vi "AWS IoT Button - Upload to S3 Bucket.vi"() -> ()   [LabVIEW 2015]
doc: "Demonstrates how to programmatically upload AWS IoT Button data to an S3 bucket."
uses:
  Core/HTTP Request/Region.ctl
  IoT/Topic Rule.ctl
  IoT/CloudWatch Alarm.ctl
  IoT/CloudWatch Metric.ctl
  IoT/DynamoDB.ctl
  IoT/DynamoDBv2.ctl
  IoT/Elasticsearch.ctl
  IoT/Firehose.ctl
  IoT/Kinesis.ctl
  IoT/Lambda.ctl
  IoT/Republish.ctl
  IoT/S3.ctl
  IoT/SNS.ctl
  IoT/SQS.ctl
  Core/HTTP Request/AWS Credentials.ctl
  IoT/IoT Session/IoT Session.lvclass
  IoT/NI_AWS_IoT.lvlib
  S3/Bucket/Bucket.lvclass
  Core/HTTP Request/HTTP Request.lvclass
panel:
  in  "Bucket Name":string
  in  "AWS IoT Button Serial Number":string
  in  "Region":T1
  in  "Secret Key":string
  in  "Access Key":string
  # "Overview: Demonstrates how to programmatically upload AWS IoT Button data to an S3 bucket.\nRequirements: NI Cloud Toolkit for AWS, a configured AWS IoT Button, and a registered Amazon AWS account\nInstructions:\n1. Specify the Access Key and Secret Key for your AWS account. You can create an account at http://aws.amazon.com.\n2. Make sure you already have an AWS IoT Button configured in the AWS IoT Management Console on the amazon website.\n3. Specify the Region under which your AWS IoT Button is configured.\n4. Specify the AWS IoT Button Serial Number.\n5. Specify the Bucket Name where you want to upload the AWS IoT Button data. Note: This bucket must already exist, and it must be in the same region as the AWS IoT Button.\n6. Run the VI.\n7. Click the AWS IoT Button. After the green light appears on the button, you can use the AWS S3 Management Console to see the button data appear as a new file in the specified S3 bucket."
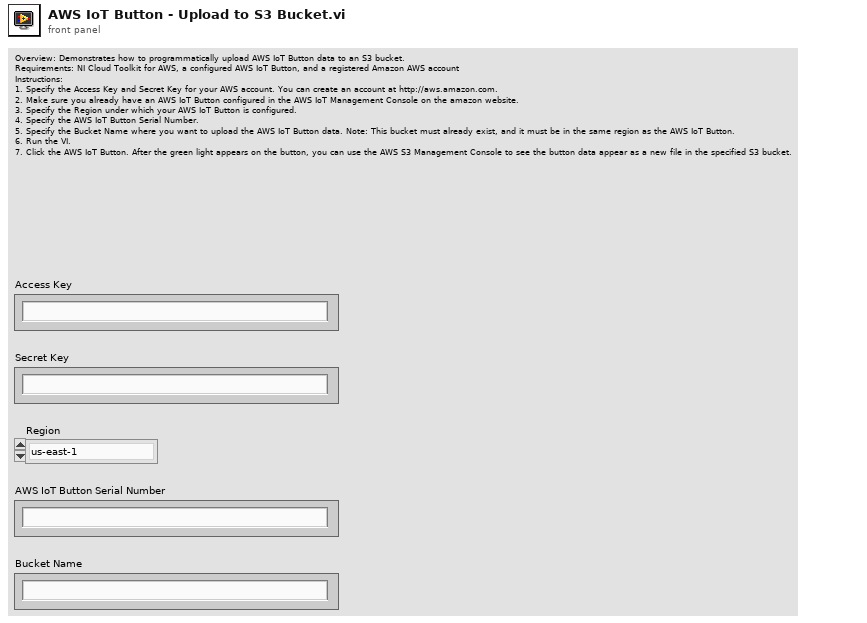
[diagram p1: front panel]
types:
  T1 = typedef "NI_AWS_Core.lvlib/HTTP Request.lvclass/Region.ctl" = enum16{"us-east-1", "us-east-2", "us-west-1", "us-west-2", "ap-northeast-1", "ap-northeast-2", "ap-southeast-1", "ap-southeast-2", "ca-central-1", "eu-central-1", "eu-west-1", "eu-west-2", "sa-east-1"}
  T2 = typedef "NI_AWS_Core.lvlib/HTTP Request.lvclass/AWS Credentials.ctl" = cluster{"Access Key":string, "Secret Key":string}
  T3 = typedef "NI_AWS_IoT.lvlib/S3.ctl" = cluster{"Bucket Name":string, "Canned ACL":string, "Key":string, "Role ARN":string}
  T4 = typedef "NI_AWS_IoT.lvlib/Topic Rule.ctl" = cluster{"CloudWatch Alarm":T5[], "CloudWatch Metric":T6[], "DynamoDB":T7[], "DynamoDBv2":T8[], "Elasticsearch":T9[], "Firehose":T10[], "Kinesis":T11[], "Lambda":T12[], "Republish":T13[], "S3":T3[], "SNS":T14[], "SQS":T15[], "AWS IoT SQL Version":string, "Description":string, "Created At":u64, "Incoming Schema ARN":string, "Outgoing Schema ARN":string, "Rule Disabled":bool, "Rule Name":string, "SQL":string, "Rule ARN":string}
  T5 = typedef "NI_AWS_IoT.lvlib/CloudWatch Alarm.ctl" = cluster{"Alarm Name":string, "Role ARN":string, "State Reason":string, "State Value":string}
  T6 = typedef "NI_AWS_IoT.lvlib/CloudWatch Metric.ctl" = cluster{"Metric Name":string, "Metric Namespace":string, "Metric Timestamp":string, "Metric Unit":string, "Metric Value":string, "Role ARN":string}
  T7 = typedef "NI_AWS_IoT.lvlib/DynamoDB.ctl" = cluster{"Hash Key Field":string, "Hash Key Type":string, "Hash Key Value":string, "Operation":string, "Payload Field":string, "Range Key Field":string, "Range Key Type":string, "Range Key Value":string, "Role ARN":string, "Table Name":string}
  T8 = typedef "NI_AWS_IoT.lvlib/DynamoDBv2.ctl" = cluster{"Role ARN":string, "Table Name":string}
  T9 = typedef "NI_AWS_IoT.lvlib/Elasticsearch.ctl" = cluster{"Endpoint":string, "ID":string, "Index":string, "Role ARN":string, "Type":string}
  T10 = typedef "NI_AWS_IoT.lvlib/Firehose.ctl" = cluster{"Delivery Stream Name":string, "Role ARN":string, "Separator":string}
  T11 = typedef "NI_AWS_IoT.lvlib/Kinesis.ctl" = cluster{"Partition Key":string, "Role ARN":string, "Stream Name":string}
  T12 = typedef "NI_AWS_IoT.lvlib/Lambda.ctl" = cluster{"Function ARN":string}
  T13 = typedef "NI_AWS_IoT.lvlib/Republish.ctl" = cluster{"Role ARN":string, "Topic":string}
  T14 = typedef "NI_AWS_IoT.lvlib/SNS.ctl" = cluster{"Message Format":string, "Role ARN":string, "Target ARN":string}
  T15 = typedef "NI_AWS_IoT.lvlib/SQS.ctl" = cluster{"Queue URL":string, "Role ARN":string, "Use Base 64":bool}
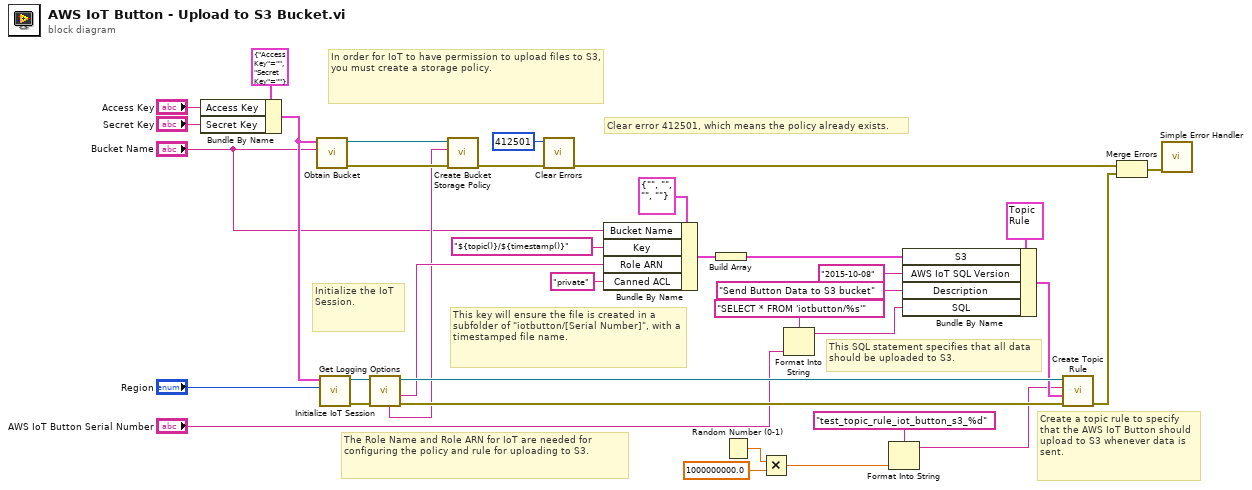
[diagram p0: block diagram]
diagram:
  # "Initialize the IoT Session."
  # "The Role Name and Role ARN for IoT are needed for configuring the policy and rule for uploading to S3."
  # "This SQL statement specifies that all data should be uploaded to S3."
  # "This key will ensure the file is created in a subfolder of \"iotbutton/[Serial Number]\", with a timestamped file name."
  # "Create a topic rule to specify that the AWS IoT Button should upload to S3 whenever data is sent."
  # "Clear error 412501, which means the policy already exists."
  # "In order for IoT to have permission to upload files to S3, you must create a storage policy."
  n1 = Bundle By Name(cluster=T2 {"Access Key"="", "Secret Key"=""} ("AWS Credentials"), "Access Key"="Access Key", "Secret Key"="Secret Key") -> (w12:T2)
  n2 = call "Obtain Bucket.vi"("Bucket name"="Bucket Name", "AWS Credentials"=w12) -> ("error out"=w24:errorcluster, "Bucket"=w19:refnum<class "Bucket.lvclass">)  [unwired: 8 in]
  n3 = call "Initialize IoT Session.vi"("Region"="Region", "AWS Credentials"=w12) -> ("error out"=w36:errorcluster, "IoT Session"=w33:refnum<class "IoT Session.lvclass">)  [unwired: 8 in]
  n4 = call "Get Logging Options.vi"("error in (no error)"=w36, "IoT Session in"=w33) -> ("error out"=w34:errorcluster, "Role ARN"=w31:string, "IoT Session out"=w32:refnum<class "IoT Session.lvclass">, "Role Name"=w18:string)  [unwired: 5 in, 1 out]
  n5 = call "Create Bucket Storage Policy.vi"("error in (no error)"=w24, "Role Name"=w18, "Bucket in"=w19) -> ("error out"=w20:errorcluster)  [unwired: 7 in, 1 out]
  n6 = call <vilib>:"Clear Errors.vi"("error in (no error)"=w20, "specific error code to clear (0: all)"=412501) -> ("error out"=w2:errorcluster)  [unwired: 4 in, 1 out]
  n7 = Bundle By Name(cluster=T3 {"Bucket Name"="", "Canned ACL"="", "Key"="", "Role ARN"=""} ("S3"), "Bucket Name"="Bucket Name", "Key"="${topic()}/${timestamp()}", "Role ARN"=w31, "Canned ACL"="private") -> (w30:T3)
  n8 = Build Array(w30) -> (w17:T3[])
  n9 = Random Number (0-1)() -> (number: 0 to 1=w5:dbl)
  n10 = Multiply(x=w5, y=1000000000.0) -> (x*y=w3:dbl)
  n11 = Format Into String(format string="SELECT * FROM 'iotbutton/%s'", "AWS IoT Button Serial Number") -> (resulting string=w25:string)  [unwired: 2 in, 1 out]
  n12 = Format Into String(format string="test_topic_rule_iot_button_s3_%d" ("Name"), w3) -> (resulting string=w21:string)  [unwired: 2 in, 1 out]
  n13 = Bundle By Name(cluster=T4 {"CloudWatch Alarm"=[], "CloudWatch Metric"=[], "DynamoDB"=[], "DynamoDBv2"=[], "Elasticsearch"=[], "Firehose"=[], "Kinesis"=[], "Lambda"=[], "Republish"=[], "S3"=[], "SNS"=[], "SQS"=[], "AWS IoT SQL Version"="", "Description"="", "Created At"=0, "Incoming Schema ARN"="", "Outgoing Schema ARN"="", "Rule Disabled"=FALSE, "Rule Name"="", "SQL"="", "Rule ARN"=""} ("Topic Rule"), "S3"=w17, "AWS IoT SQL Version"="2015-10-08", "Description"="Send Button Data to S3 bucket", "SQL"=w25) -> (w27:T4)
  n14 = call "Create Topic Rule.vi"("error in (no error)"=w34, "Topic Rule"=w27, "Rule Name"=w21, "IoT Session in"=w32) -> ("error out"=w23:errorcluster)  [unwired: 6 in, 1 out]
  n15 = Merge Errors(w2, w23) -> (w14:errorcluster)
  n16 = call <vilib>:"Simple Error Handler.vi"("error in (no error)"=w14) -> ()  [unwired: 4 in, 5 out]
